vi "SubVI_Ger_Funcoes.vi"(3 "Tensão (Vp)":dbl, 4 "Frequencia (Hz)":dbl, 5 "Gerador de Funções":refnum<visa-resource-name>="GPIB0::10::INSTR") -> (0 "Tensão atual":dbl, 1 "Freq_Atual":dbl, 2 "VISA resource name out":refnum<visa-resource-name>)   [LabVIEW 2018]
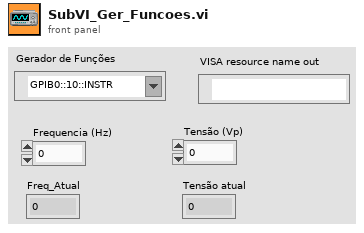
[diagram p1: front panel]
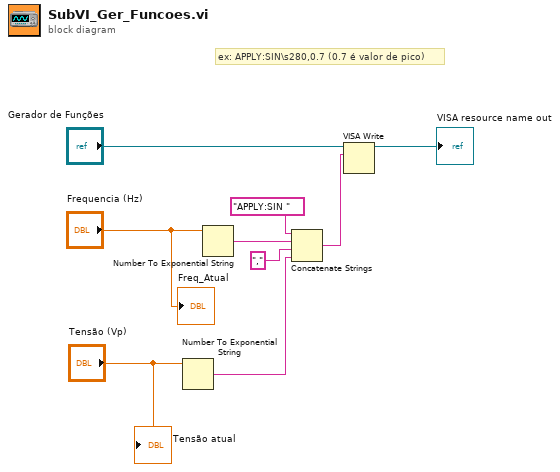
[diagram p0: block diagram]
diagram:
  # "ex: APPLY:SIN\\s280,0.7 (0.7 é valor de pico)"
  n1 = Number To Exponential String(number="Tensão (Vp)") -> (E-format string=w7:string)  [unwired: 3 in]
  n2 = Number To Exponential String(number="Frequencia (Hz)") -> (E-format string=w9:string)  [unwired: 3 in]
  n3 = Concatenate Strings("APPLY:SIN " ("write buffer"), w9, "," ("string"), w7) -> (w5:string)
  n4 = VISA Write(VISA resource name="Gerador de Funções", write buffer=w5) -> (VISA resource name out=→"VISA resource name out":refnum<visa-resource-name>)  [unwired: 1 in, 2 out]
  "Freq_Atual" <- "Frequencia (Hz)"
  "Tensão atual" <- "Tensão (Vp)"
